vi "Dashboard Main.vi"() -> ()   [LabVIEW 2014]
uses:
  <vilib>/event_ctls.llb/eventvkey.ctl
  <vilib>/Rock Robotics/WPI/Dashboard/WPI_DashboardLogging Global.vi
  <vilib>/Utility/config.llb/Write Key (String).vi
  <vilib>/Utility/config.llb/Write Key (I32).vi
  Variables/Config_Global.vi
  <vilib>/Utility/config.llb/NI_LVConfig.lvlib
panel:
  out "error out 4":errorcluster
  out "error out 3":errorcluster
  out "error out 2":errorcluster
  out "error out":errorcluster
  in  "Rec Mode":enum32{"Stop", "Record", "Playback"}(radio)
  out "Camera Image":T1(plugin-control)
  out "Boolean":bool
  in  "TCP":refnum<k5>
  in  "Vision":u16(ring) items=["Camera Off", "USB Camera SW", "USB Camera HW", "IP Camera"]
  out "Camera IP":string
  out "Image Message":string="Timeout in Camera Communications"
  in  "Dashboard Tab":T2(tab)
  in  "Camera Settings":T3={"Frame Rate"=30, "Compression"=30, "Size"=1} {"Frame Rate" scale=1.0..30.0; "Size" items=["640x480", "320x240", "160x120"]}
  out "MotorChart R":cluster{"Numeric":dbl, "Numeric":dbl}(graph)
  out "MotorChart L":T4(graph)
  out "MotorSliders R":cluster{"MotorSlide1":dbl, "MotorSlide2":dbl} {"MotorSlide2" scale=-1.0..1.0 scale format="%#_2e"; "MotorSlide1" scale=-1.0..1.0 scale format="%#_2e"}
  out "MotorSliders L":T5 {"MotorSlide4 2" scale=0.0..14.0 scale format="%#_2e"; "MotorSlide2" scale=-1.0..1.0 scale format="%#_2e"; "MotorSlide1" scale=-1.0..1.0 scale format="%#_2e"}
  out "Gyro":dbl(knob) scale=0.0..360.0
  out "JS1 Z":dbl(slide) scale=-1.0..1.0 scale format="%#_2e"
  out "JS1 Graph":cluster{"X":dbl, "Y":dbl}[](graph)
  out "JS1 Buttons":T6
  out "JS2 Z":dbl(slide) scale=-1.0..1.0 scale format="%#_2e"
  out "JS2 Graph":cluster{"X":dbl, "Y":dbl}[](graph)
  out "JS2 Buttons":T6
  out "Mode":T7(ring)=enum."Auto Disabled"
  in  "DB Camera Config":bool
  out "fps":dbl format="%#.1g"
  out "Mbps":dbl format="%#.1g"
  out "Mbps 2":bool
  in  "DB/String 9":string
  in  "DB/String 8":string
  in  "DB/String 7":string
  in  "DB/String 6":string
  in  "DB/String 5":string
  in  "DB/String 4":string
  in  "DB/String 3":string
  in  "DB/String 2":string
  in  "DB/String 1":string
  in  "DB/String 0":string
  in  "DB/Slider 0":dbl(slide) scale=0.0..5.0
  in  "DB/Slider 1":dbl(slide) scale=0.0..5.0
  in  "DB/Slider 2":dbl(slide) scale=0.0..5.0
  in  "DB/Slider 3":dbl(slide) scale=0.0..5.0
  out "DB/LED 3":bool
  out "DB/LED 2":bool
  out "DB/LED 1":bool
  out "DB/LED 0":bool
  in  "DB/Button 3":bool
  in  "DB/Button 2":bool
  in  "DB/Button 1":bool
  in  "DB/Button 0":bool caption="New Name"
  in  "Test Slider":dbl(slide) scale=0.0..100.0 scale format="%#_3g"
  in  "On/Off":bool caption="Solenoid"
  in  "Test Name":u16(ring) items=["Select the test to run...", "Example Test", "-------------------------------", "List of tests is built in robot code.", "Replace with your own automated tests."]
  in  "Test Tree":string(tree)
  in  "Motor":cluster{"Value":dbl, "Enable":bool} {"Value" scale=-1.0..1.0 scale format="%#_3g"}
  out "Progress":T8 {"Test Progress" scale=0.0..100.0}
  in  "Rev/Fwd":cluster{"Forward":bool, "Reverse":bool}
  in  "Test Ring":u16(ring) items=["Monochrome", "Color"]
  in  "Listbox":i32(listbox)
  out "Tree":string(tree)
  in  "Tab Control 2":T9(tab)
  in  "Pod 0":T10
  in  "Pod 1":T10
  in  "Pod 2":T10
  in  "Pod 3":T10
  in  "General":T11
  out "error out":errorcluster
  # "Left"
  # "Front"
  # "Right"
  # "Battery"
  # "This tab is a great place for autonomous settings and robot-specific values.\nPlace controls and indicators inside this tab and match name to\nDashboard Variables on robot. You can also delete this comment."
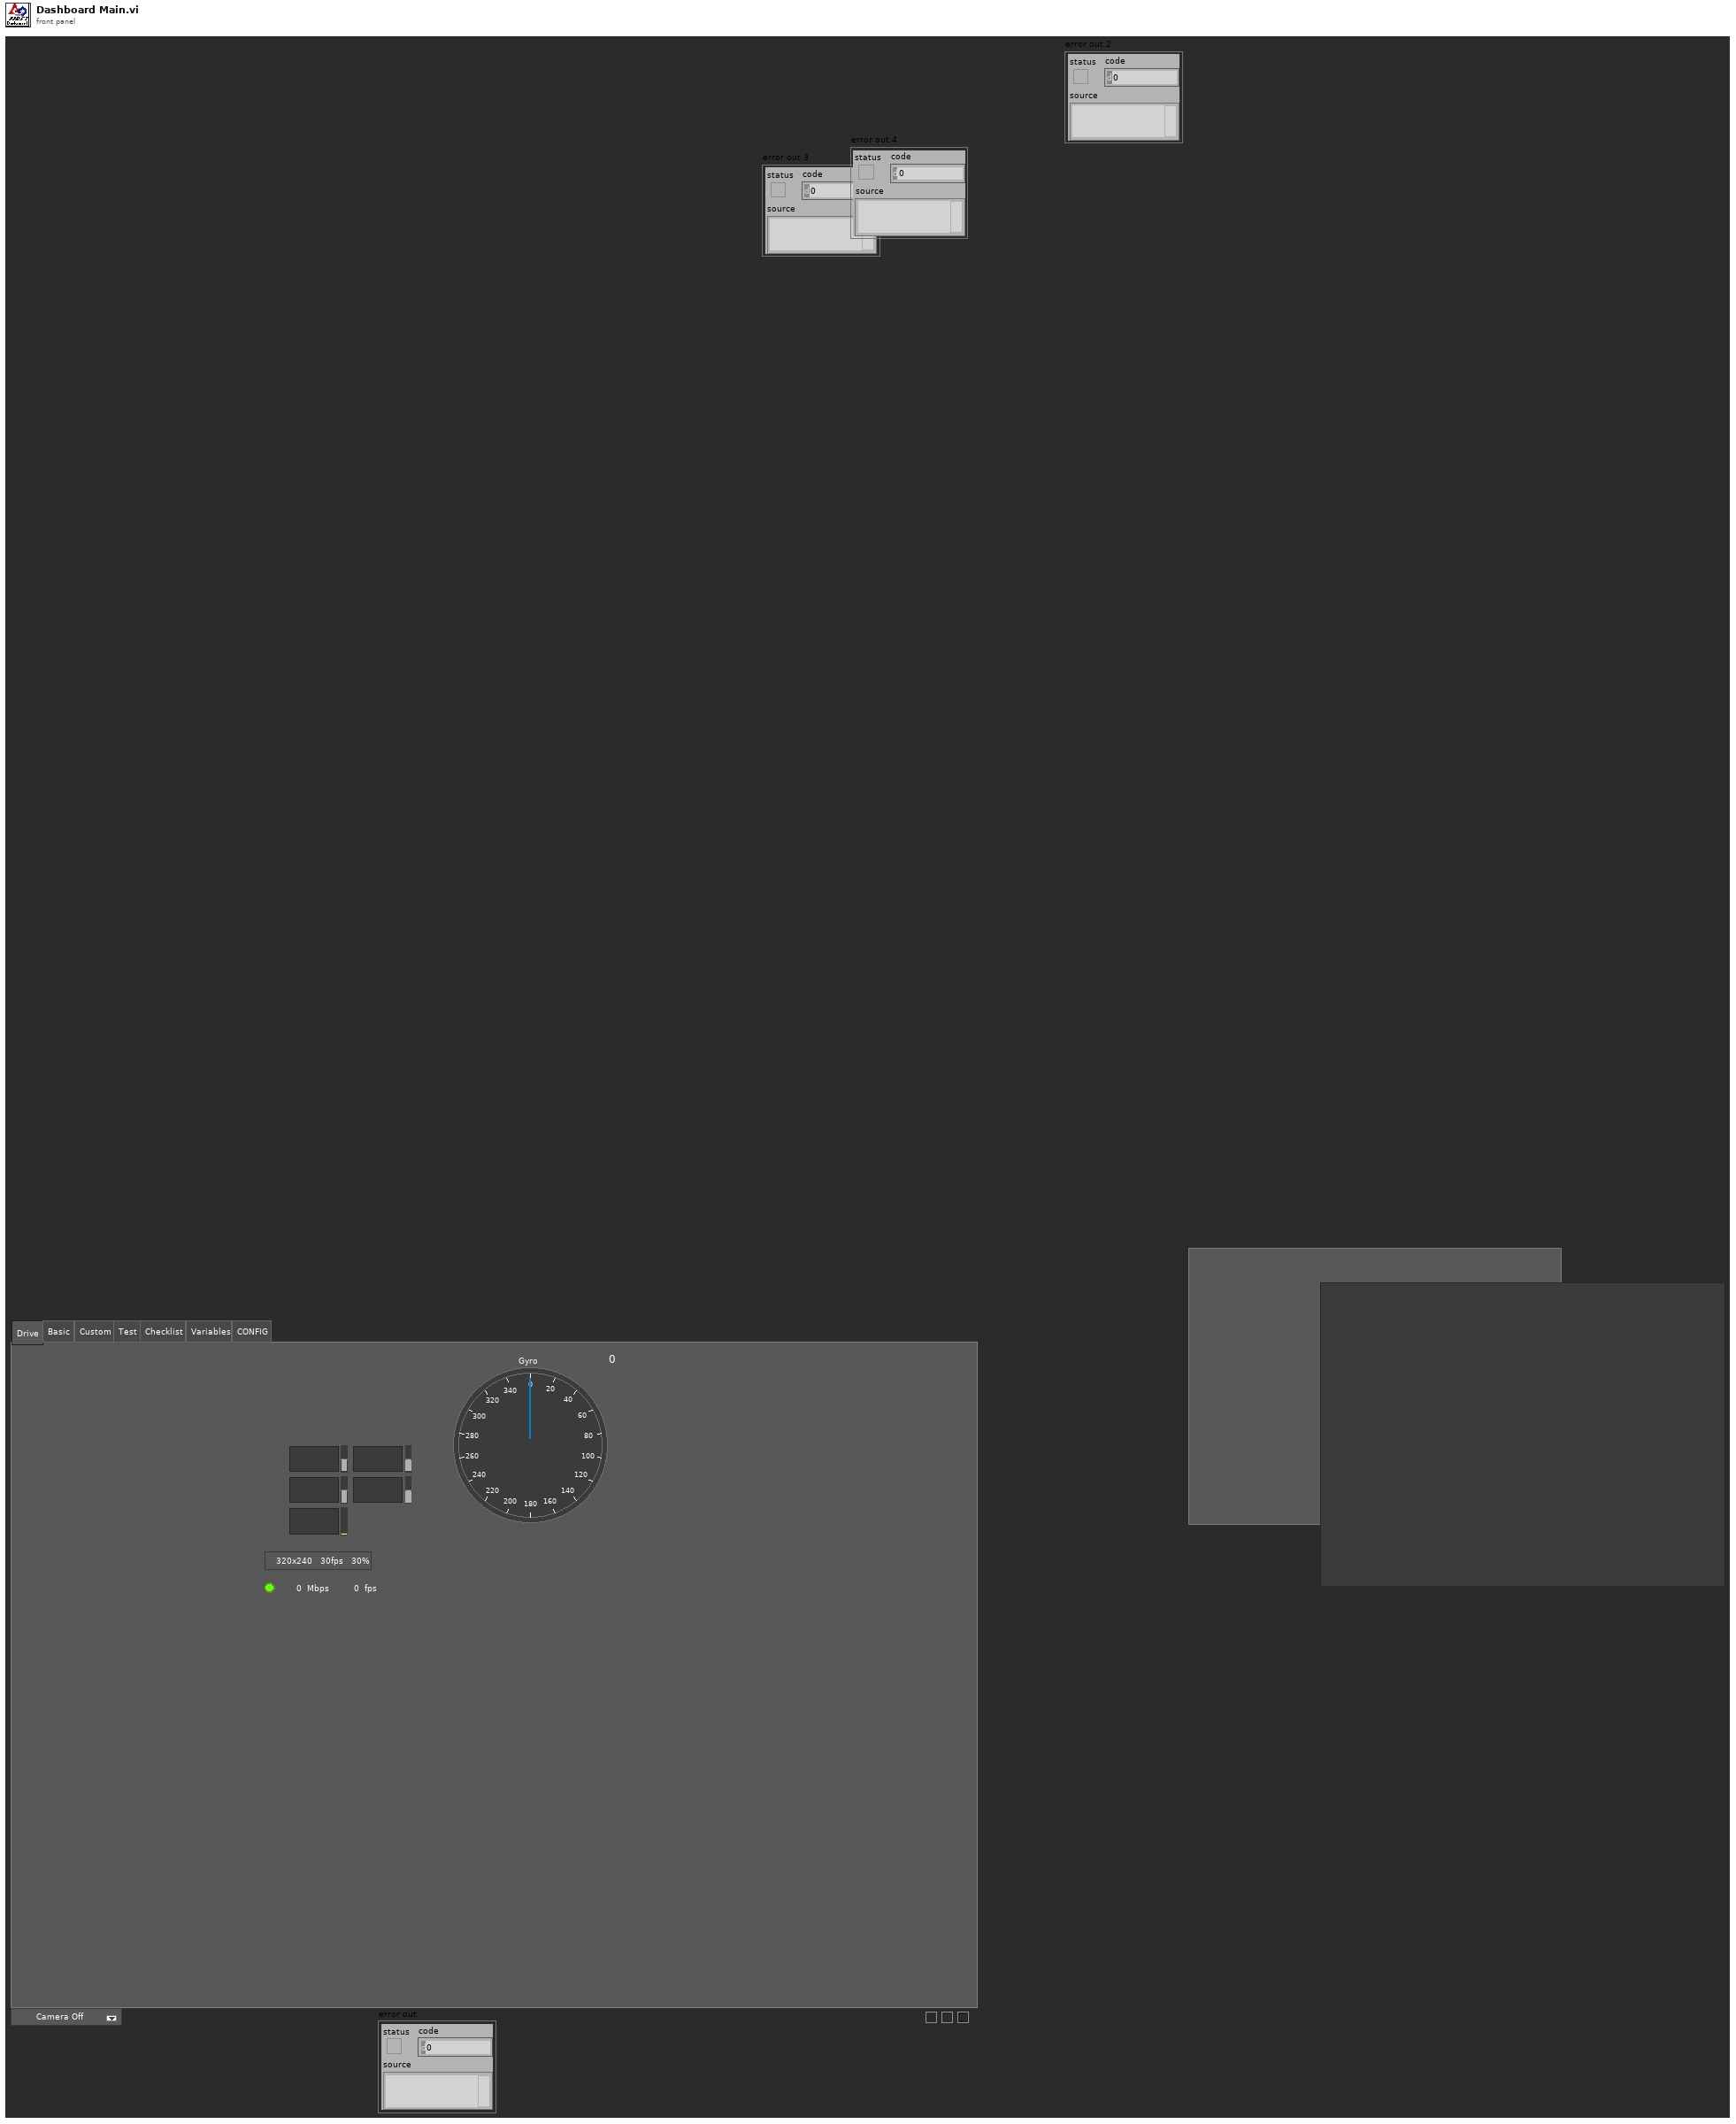
[diagram p1: front panel]
types:
  T1 = typedef "IMAQ Image.ctl" = refnum<image>
  T2 = enum32{"Drive", "Basic", "Custom", "Test", "Checklist", "Variables", "CONFIG"}
  T3 = cluster{"Frame Rate":i32, "Compression":i32, "Size":u16}
  T4 = cluster{"Numeric":dbl, "Numeric":dbl, "Battery V":dbl}
  T5 = cluster{"MotorSlide1":dbl, "MotorSlide2":dbl, "MotorSlide4 2":dbl}
  T6 = cluster{bool, bool, bool, bool, bool, bool, bool, bool, bool, bool, bool, bool}
  T7 = enum8{"Tele-Op Disabled", "Tele-Op Enabled", "Auto Disabled", "Auto Enabled", "Test Disabled", "Test Enabled", "Disconnected", "No Code", "E-Stop"}
  T8 = cluster{"Test Progress":u8, "Test Progress Text":string}
  T9 = enum32{"Pod 0", "Pod 1", "Pod 2", "Pod 3", "General"}
  T10 = cluster{"Drive":cluster{"DriveEncoder_CPfoot":dbl, "DriveEncoder_Location":string, "DriveEncoder_RoboRIO_PinA":i32, "DriveEncoder_RoboRIO_PinB":i32, "DriveEncoder_Invert?":bool, "DriverMotor_PID_P":dbl, "DriverMotor_PID_I":dbl, "DriverMotor_PID_D":dbl, "DriveMotor_CANorPWN_Channel":i32, "DriveMotor_Invert?":bool, "DriveMotor_IsCanSRX?":bool, "DriveMotor_MaxOutput":dbl, "DriveMotor_mINOutput":dbl}, "Turret":cluster{"TurretEncoder_Invert?":bool, "TurretEncoder_ZeroPosVolts":dbl, "TurretEncoder_Location":string, "TurretEncoder_RIO_AnalogChannel":dbl, "TurretMotor_Invert?":bool, "TurretMotor_PID_P":dbl, "TurretMotor_PID_I":dbl, "TurretMotor_PID_D":dbl, "TurretMotor_CANorPWN_Channel":dbl, "TurretMotor_IsCanSRX?":bool, "TurretMotor_MaxOutput?":dbl, "TurretMotor_MinOutput":dbl}, "Misc":cluster{"PodPosition_X":dbl, "PodPosition_Y":dbl, "PDP_Channel_Drive":i32, "PDP_Channel_Turret":i32}, "error out":errorcluster, "Warning":string}
  T11 = cluster{"PodCount":dbl, "PDP_CAN_ID":i32, "PCM_CAN_ID":i32, "BaseRobotMass":dbl, "Warning":string, "error out":errorcluster}
  T12 = enum32{"Drive", "Basic", "Custom", "Test", "Checklist", "Variables"}
  T13 = typedef "Image Type" = u32
  T14 = cluster{"Camera Image":refnum<vi>, "Dashboard Tab":refnum<vi>, "Boolean":refnum<vi>, "Vision":refnum<vi>, "Rec Mode":refnum<vi>, "Test Slider":refnum<vi>, "On/Off ":refnum<vi>, "Test Ring":refnum<vi>, "Rev/Fwd":refnum<vi>, "Test Name":refnum<vi>, "Motor":refnum<vi>, "Progress":refnum<vi>, "CheckList":refnum<vi>, "Tree":refnum<vi>, "Test Tree":refnum<vi>}
  T15 = cluster{"Error Strings":string, "Disable Counts":cluster{u16, u16}, "Rail Faults":cluster{u16, u16, u16}, "Robot IP":string, "DB Mode":u8, "Event Info":cluster{"Name":string, "Type":u8, "Number":u16, "Replay":u8}, "Camera Addr":string}
  T16 = cluster{"Storage":cluster{"Disk Free":u64, "RAM Block":u32, "RAM free":u32}, "CPU Utilization":cluster{"CPU % ISR":sgl, "CPU % Time Crit":sgl, "CPU % Timed Str":sgl, "CPU % High":sgl, "CPU % Above":sgl, "CPU % Normal":sgl, "CPU % Low":sgl}, "CAN":cluster{"% Bus Utilization":sgl, "Bus Off Cnt":u32, "TX_FIFO Full Cnt":u32, "Receive Error Cnt":u8, "Transmit Error Cnt":u8}, "HID":cluster{"HID Outputs":u32, "Rumble Low":u16, "Rumble High":u16}[]}
  T17 = cluster{"Status bits":cluster{"Test Mode":bool, "Autonomous":bool, "Enabled":bool, "Code Start":bool, "Brownout":bool, "Reserved 2":bool, "Reserved 3":bool, "E-Stop":bool}, "Code Trace":cluster{"Disabled":bool, "TeleOp":bool, "Auto":bool, "Test":bool}, "Controller Type":enum16{"unknown", "cRIO", "roboRio"}, "Code?":enum16{"unknown", "noCode", "code"}, "Battery V":dbl}
  T18 = cluster{"Control Bits":cluster{"TestMode":bool, "Autonomous":bool, "Enabled":bool, "FMS Present":bool, bool, bool, bool, "E-Stop":bool}, "Team Station ":u8, "Countdown":sgl, "Joystick Values":cluster{"Axes":dbl[], "Buttons":bool[], "POVs":i16[]}[]}
  T19 = cluster{"Axes":dbl[], "Buttons":bool[], "POVs":i16[]}[]
  T20 = cluster{"Axes":dbl[], "Buttons":bool[], "POVs":i16[]}
  T21 = cluster{"Buttons[0]":bool, "Buttons[1]":bool, "Buttons[2]":bool, "Buttons[3]":bool, "Buttons[4]":bool, "Buttons[5]":bool, "Buttons[6]":bool, "Buttons[7]":bool, "Buttons[8]":bool, "Buttons[9]":bool, "Buttons[10]":bool, "Buttons[11]":bool}
  T22 = typedef "NI_LVConfig.lvlib/Config Data RefNum.ctl" = refnum<k1>
  T23 = cluster{"Operation":enum16{"Update", "Clear"}, "Color Box":u32}[]
  T24 = typedef "eventvkey.ctl" = enum16{"ASCII", "Enter", "Return", "Shift", "Ctrl", "Alt", "Cmd", "Opt", "Caps", "NumLock", "Clear", "Break", "Up", "Down", "Left", "Right", "Insert", "Delete", "Home", "End", "PageUp", "PageDown", "Escape", "Help", "Pause", "ScrollLock", "F1", "F2", "F3", "F4", "F5", "F6", "F7", "F8", "F9", "F10", "F11", "F12", "F13", "F14", "F15", "F16", "F17", "F18", "F19", "F20", "F21", "F22", "F23", "F24", "Play", "VolumeUp", "VolumeDown", "Mute", "Two Byte Char"}
  T25 = cluster{"Image Size":bool, "Image Type":bool, "Pixel Value":bool, "ROI Information":bool, "Zoom Factor":bool}
  T26 = enum8{"Enabled", "Disabled", "Disabled and Grayed Out"}
  T27 = cluster{"Operation":enum16{"Update", "Clear"}, "Color Box":u32}
  T28 = cluster{"DriveEncoder_CPfoot":dbl, "DriveEncoder_Location":string, "DriveEncoder_RoboRIO_PinA":i32, "DriveEncoder_RoboRIO_PinB":i32, "DriveEncoder_Invert?":bool, "DriverMotor_PID_P":dbl, "DriverMotor_PID_I":dbl, "DriverMotor_PID_D":dbl, "DriveMotor_CANorPWN_Channel":i32, "DriveMotor_Invert?":bool, "DriveMotor_IsCanSRX?":bool, "DriveMotor_MaxOutput":dbl, "DriveMotor_mINOutput":dbl}
  T29 = cluster{"TurretEncoder_Invert?":bool, "TurretEncoder_ZeroPosVolts":dbl, "TurretEncoder_Location":string, "TurretEncoder_RIO_AnalogChannel":dbl, "TurretMotor_Invert?":bool, "TurretMotor_PID_P":dbl, "TurretMotor_PID_I":dbl, "TurretMotor_PID_D":dbl, "TurretMotor_CANorPWN_Channel":dbl, "TurretMotor_IsCanSRX?":bool, "TurretMotor_MaxOutput?":dbl, "TurretMotor_MinOutput":dbl}
  T30 = cluster{"PodPosition_X":dbl, "PodPosition_Y":dbl, "PDP_Channel_Drive":i32, "PDP_Channel_Turret":i32}
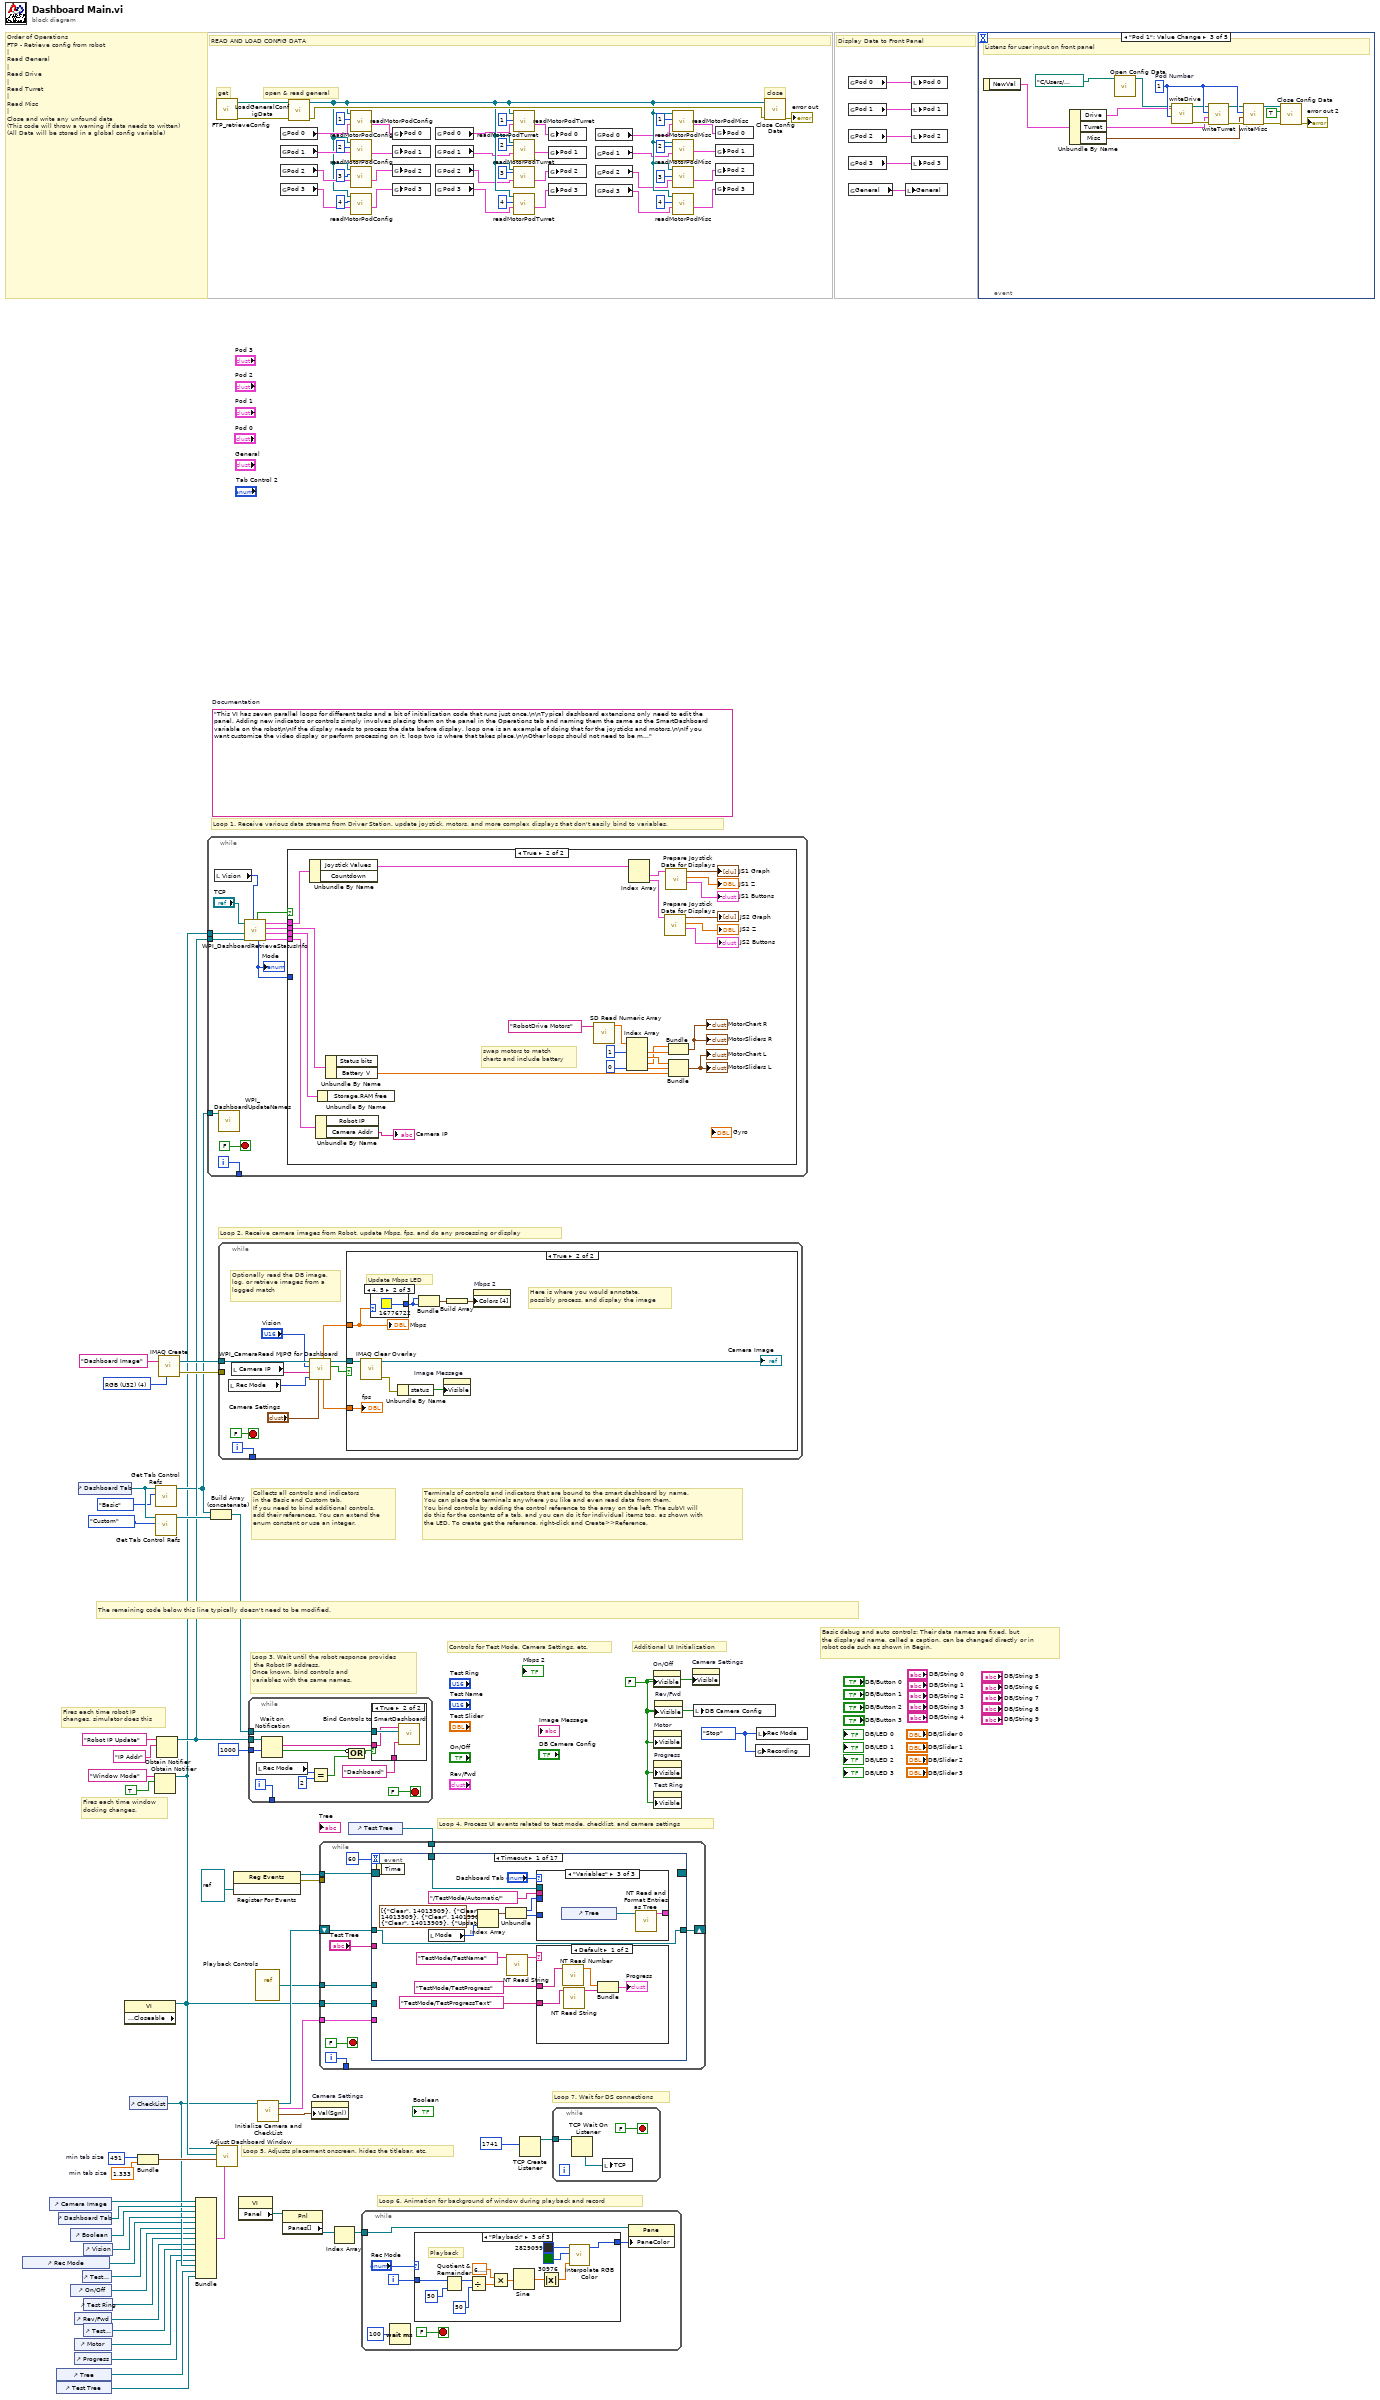
[diagram p0: block diagram]
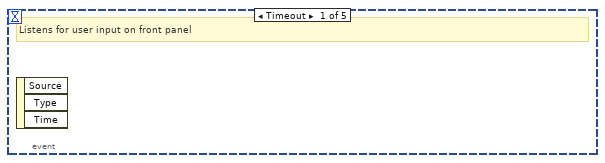
[diagram p2: hidden frame]
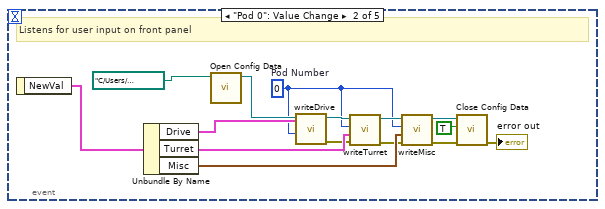
[diagram p3: hidden frame]
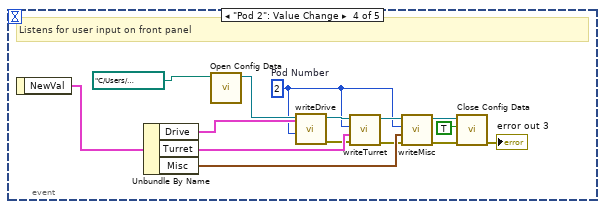
[diagram p4: hidden frame]
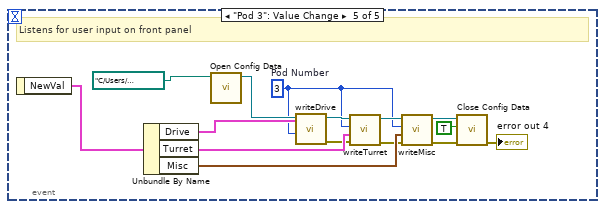
[diagram p5: hidden frame]
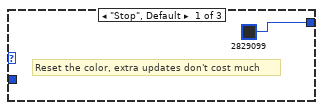
[diagram p7: hidden frame]
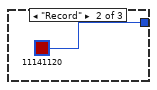
[diagram p8: hidden frame]
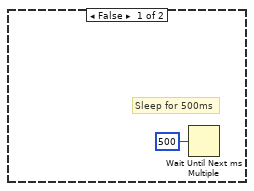
[diagram p10: hidden frame]
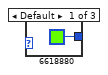
[diagram p11: hidden frame]
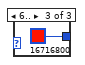
[diagram p12: hidden frame]
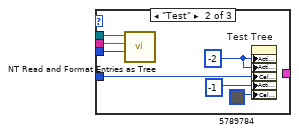
[diagram p14: hidden frame]
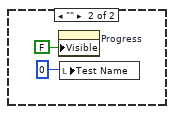
[diagram p15: hidden frame]
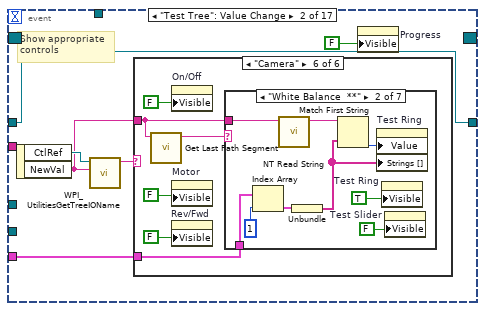
[diagram p16: hidden frame]
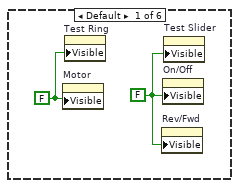
[diagram p17: hidden frame]
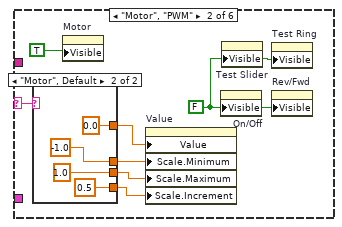
[diagram p18: hidden frame]
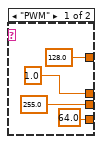
[diagram p19: hidden frame]
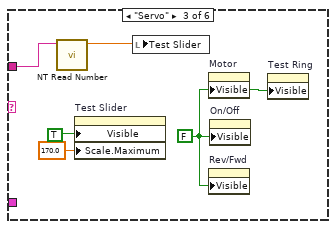
[diagram p20: hidden frame]
diagram:
  w70 = 491  # min tab size
  w69 = 1.333  # min tab size
  w78 = enum32{"Stop", "Record", "Playback"}."Stop" ("Rec Mode")
  w52 = FALSE ("Visible")
  (unwired) "This VI has seven parallel loops for different tasks and a bit of initialization code that runs just once.\n\nTypical dashboard extensions only need to edit the panel. Adding new indicators or controls simply involves placing them on the panel in the Operations tab and naming them the same as the SmartDashboard variable on the robot\n\nIf the display needs to process the data before display, loop one is an example of doing that for the joysticks and motors.\n\nIf you want customize the video display or perform processing on it, loop two is where that takes place.\n\nOther loops should not need to be modified. They are pretty standard, and document the task they perform."  # Documentation
  w98 = T13 4 items=["Grayscale (U8)", "Grayscale (I16)", "Grayscale (SGL)", "Complex (CSG)", "RGB (U32)", "HSL (U32)", "RGB (U64)"] ("Image Type")
  # "Display Data to Front Panel"
  # "Order of Operations\nFTP - Retrieve config from robot\n|\nRead General\n|\nRead Drive\n|\nRead Turret\n|\nRead Misc\n|\nClose and write any unfound data\n(This code will throw a warning if data needs to written)\n(All Data will be stored in a global config variable)"
  # "READ AND LOAD CONFIG DATA"
  # "open & read general"
  # "get"
  # "close"
  # "Loop 7. Wait for DS connections"
  # "Basic debug and auto controls: Their data names are fixed, but\nthe displayed name, called a caption, can be changed directly or in\nrobot code such as shown in Begin."
  # "Controls for Test Mode, Camera Settings, etc."
  # "Additional UI Initialization"
  # "Loop 6. Animation for background of window during playback and record"
  # "Fires each time robot IP\nchanges, simulator does this"
  # "Fires each time window\ndocking changes."
  # "Collects all controls and indicators\nin the Basic and Custom tab.\nIf you need to bind additional controls,\nadd their references. You can extend the\nenum constant or use an integer."
  # "The remaining code below this line typically doesn't need to be modified."
  # "Loop 4. Process UI events related to test mode, checklist, and camera settings"
  # "Terminals of controls and indicators that are bound to the smart dashboard by name.\nYou can place the terminals anywhere you like and even read data from them.\nYou bind controls by adding the control reference to the array on the left. The subVI will\ndo this for the contents of a tab, and you can do it for individual items too, as shown with\nthe LED. To create get the reference, right-click and Create>>Reference."
  # "Loop 3. Wait until the robot response provides\n the Robot IP address.\nOnce known, bind controls and\nvariables with the same names."
  # "Loop 5. Adjusts placement onscreen, hides the titlebar, etc."
  # "Loop 1. Receive various data streams from Driver Station, update joystick, motors, and more complex displays that don't easily bind to variables."
  # "Loop 2. Receive camera images from Robot, update Mbps, fps, and do any processing or display"
  n1 = control-ref of="Rec Mode"() -> (w58:refnum<vi>)
  n2 = control-ref of="Camera Image"() -> (w73:refnum<vi>)
  n3 = control-ref of="Tree"() -> (w62:refnum<vi>)
  n4 = control-ref of="Test Tree"() -> (w61:refnum<vi>)
  n5 = control-ref of="Dashboard Tab"() -> (w72:refnum<vi>)
  n6 = control-ref of="Boolean"() -> (w67:refnum<vi>)
  n7 = control-ref of="On/Off"() -> (w56:refnum<vi>)
  n8 = control-ref of="Progress"() -> (w53:refnum<vi>)
  n9 = control-ref of="Rev/Fwd"() -> (w54:refnum<vi>)
  n10 = control-ref of="Motor"() -> (w59:refnum<vi>)
  n11 = control-ref of="Dashboard Tab"() -> (w76:refnum<vi>)
  n12 = control-ref of="Test Slider"() -> (w57:refnum<vi>)
  n13 = control-ref of="Vision"() -> (w71:refnum<vi>)
  n14 = control-ref of="Test Ring"() -> (w55:refnum<vi>)
  n15 = control-ref of="Test Name"() -> (w60:refnum<vi>)
  n16 = property class="VI" props=["Front Panel.Closeable"]() -> (reference out=w77:refnum<vi>)  [unwired: 2 in, 2 out]
  n17 = control-ref of="CheckList"() -> (w63:refnum<vi>)
  n18 = Bundle("min tab size"=w70, "min tab size"=w69) -> (w68:cluster{"min tab size":i32, "min tab size":dbl})  [unwired: 1 in]
  n19 = Obtain Notifier(name (unnamed)="Window Mode", notification data type=TRUE) -> (notifier out=w49:refnum<notifier>)  [unwired: 2 in, 2 out]
  n20 = call <vilib>:"Get Tab Control Refs.vi"("Page Index"=T12."Basic" ("Dashboard Tab"), "TabControl in"=w76) -> ("ControlsOnPage"=w50:refnum<vi>[])  [unwired: 9 in]
  n21 = call <vilib>:"Get Tab Control Refs.vi"("Page Index"=T12."Custom" ("Dashboard Tab"), "TabControl in"=w76) -> ("ControlsOnPage"=w75:refnum<vi>[])  [unwired: 9 in]
  n22 = Obtain Notifier(name (unnamed)="Robot IP Update", notification data type="IP Addr" ("name (unnamed)")) -> (notifier out=w51:refnum<notifier>)  [unwired: 2 in, 2 out]
  n23 = call "IMAQ Create"("Image Name"="Dashboard Image", "Image Type"=w98) -> ("New Image"=w96:T1, "error out"=w95:errorcluster)  [unwired: 2 in, 1 out]
  n24 = Bundle("Camera Image"=w73, "Dashboard Tab"=w72, "Boolean"=w67, "Vision"=w71, "Rec Mode"=w58, "Test Slider"=w57, "On/Off"=w56, "Test Ring"=w55, "Rev/Fwd"=w54, "Test Name"=w60, "Motor"=w59, "Progress"=w53, "CheckList"=w63, "Tree"=w62, "Test Tree"=w61) -> (w64:T14)  [unwired: 1 in]
  n25 = while {
    tunnel: [w110] -> _
    tunnel: w51 -> [w104]
    tunnel: w50 -> [w103]
    tunnel: w49 -> [w99]
    i -> [w110]
    stop <- FALSE stop-if-true
    n26 = local read "Vision"() -> (w101:u16)
    n27 = call <vilib>:"WPI_DashboardUpdateNames.vi"("Controls on Tab"=w103) -> ()  [unwired: 11 in]
    n28 = call <vilib>:"WPI_DashboardRetrieveStatusInfo.vi"("Vision"=w101, "Binding Refnum"=w104, "Window Mode Notifier"=w99, "TCP Cnx"="TCP") -> ("Power and Errors"=w105:T15, "Robot Metrics"=w108:T16, "Status Info"=w109:T17, "Control Info"=w106:T18, "Robot Mode"=w102:T7, "Process?"=w107:bool)  [unwired: 2 in]
    "Mode" <- w102
    n29 = case shown="True" w107 {
      tunnel: w109 -> [_ w136]
      tunnel: w108 -> [_ w135]
      tunnel: w106 -> [_ w134]
      tunnel: w105 -> [_ w133]
      tunnel: w102 -> [_ _]
      frame False {
      }
      frame True {
        # "swap motors to match\ncharts and include battery"
        n30 = Unbundle By Name(w134) -> ("Joystick Values"=w121:T19)  [unwired: 1 out]
        n31 = Unbundle By Name(w133) -> ("Camera Addr"=→"Camera IP":string)  [unwired: 1 out]
        n32 = Unbundle By Name(w135) -> ()  [unwired: 1 out]
        n33 = Unbundle By Name(w136) -> ("Battery V"=w122:dbl)  [unwired: 1 out]
        n34 = call <vilib>:"SD Read Numeric Array.vi"("Name"="RobotDrive Motors") -> ("Numeric Array"=w124:dbl[])  [unwired: 8 in, 2 out]
        n35 = Index Array(array=w124, index #1=1, index #4=0) -> (element #1=w128:dbl, element #2=w129:dbl, element #3=w127:dbl, element #4=w132:dbl)  [unwired: 2 in]
        n36 = Index Array(array=w121) -> (element #1=w120:T20, element #2=w115:T20)  [unwired: 2 in]
        n37 = call "Prepare Joystick Data for Displays.vi"("Joystick Values"=w115) -> ("Buttons"=→"JS2 Buttons":T21, "Z Axis"=→"JS2 Z":dbl, "Cartesian Data"=→"JS2 Graph":cluster{"X axis":dbl, "X axis":dbl}[])  [unwired: 8 in]
        n38 = call "Prepare Joystick Data for Displays.vi"("Joystick Values"=w120) -> ("Buttons"=→"JS1 Buttons":T21, "Z Axis"=→"JS1 Z":dbl, "Cartesian Data"=→"JS1 Graph":cluster{"X axis":dbl, "X axis":dbl}[])  [unwired: 8 in]
        n39 = Bundle("Numeric"=w127, "Numeric"=w128) -> (→"MotorChart R" →"MotorSliders R":cluster{"Numeric":dbl, "Numeric":dbl})  [unwired: 1 in]
        n40 = Bundle("Numeric"=w129, "Numeric"=w132, "Battery V"=w122) -> (→"MotorChart L" →"MotorSliders L":T4)  [unwired: 1 in]
      }
    }
  }
  n41 = Build Array (concatenate)(w50, w75) -> (w74:refnum<vi>[])
  n42 = call "FTP_retrieveConfig.vi"() -> ("error out"=w45:errorcluster, "local path"=w46:path)  [unwired: 10 in]
  n43 = call "Adjust Dashboard Window.vi"("Sizing Refnums"=w64, "Size Constraints"=w68, "VI"=w77, "Notifier in"=w49) -> ()  [unwired: 8 in]
  n44 = while {
    tunnel: w96 -> [w145]
    tunnel: w95 -> [_]
    tunnel: [w146] -> _
    i -> [w146]
    stop <- FALSE stop-if-true
    # "Optionally read the DB image,\nlog, or retrieve images from a\nlogged match"
    n45 = local read "Rec Mode"() -> (w139:enum32{"Stop", "Record", "Playback"})
    n46 = local read "Camera IP"() -> (w137:string)
    n47 = call <vilib>:"WPI_CameraRead MJPG for Dashboard.vi"("Camera Settings"="Camera Settings", "Rec Mode"=w139, "Camera IP"=w137, "Camera Mode"="Vision", "Refnum in"=w145) -> ("Active"=w143:bool, "Refnum out"=w144:T1, "FPS"=w142:dbl, "Bandwidth (Mbps)"=w141:dbl)  [unwired: 3 in]
    n48 = case shown="True" w143 {
      tunnel: w144 -> [_ w152]
      tunnel: w141 -> [_ w151]
      tunnel: w142 -> [_ w149]
      frame False {
        # "Sleep for 500ms"
        n49 = Wait Until Next ms Multiple(millisecond multiple=u32 500) -> ()  [unwired: 1 out]
      }
      frame True {
        # "Here is where you would annotate,\npossibly process, and display the image"
        # "Update Mbps LED"
        n50 = call "IMAQ Clear Overlay"("Image"=w152) -> ("error out"=w156:errorcluster, "Image Out"=→"Camera Image":T1)  [unwired: 2 in, 7 out]
        n51 = case shown="4, 5" w151 {
          tunnel: [u32 6618880 ("Color Box") u32 16776722 ("Color Box") u32 16716800 ("Color Box")] -> w153
          frame Default {
          }
          frame 4, 5 {
          }
          frame 6.. {
          }
        }
        n52 = Unbundle By Name(w156) -> ("status"=w157:bool)
        n53 = Bundle("Color Box"=w153, "Color Box"=w153) -> (w155:cluster{"Color Box":u32, "Color Box":u32})  [unwired: 1 out]
        n54 = property on="Image Message" class="Str"("Visible"=w157) -> ()  [unwired: 2 in, 2 out]
        n55 = Build Array(w155) -> (w154:cluster{"Color Box":u32, "Color Box":u32}[])
        n56 = property on="Mbps 2" class="Bool (strict)"("Colors [4]"=w154) -> ()  [unwired: 2 in, 2 out]
        "Mbps" <- w151
        "fps" <- w149
      }
    }
  }
  n57 = register-events(refnum<vi> refnum) -> (reference out=w82:refnum<event-registration>, error out=w81:errorcluster)  [unwired: 2 in]
  n58 = property class="VI"() -> ("Panel"=w85:refnum<vi>)  [unwired: 2 in, 2 out]
  n59 = while {
    tunnel: w74 -> [w172]
    tunnel: w51 -> [w170]
    tunnel: [w168] -> _
    tunnel: u32 1000 ("milliseconds to wait") -> [w167]
    i -> [w168]
    stop <- FALSE stop-if-true
    n60 = local read "Rec Mode"() -> (w163:enum32{"Stop", "Record", "Playback"})
    n61 = Wait on Notification(notifier=w170, timeout in ms (-1)=w167) -> (notification=w169:string, timed out?=w165:bool)  [unwired: 2 in, 2 out]
    n62 = Equal?(x=w163, y=u16 2 ("Rec Mode")) -> (x = y?=w164:bool)
    n63 = Compound Arithmetic op=OR(invert w165, w164) -> (w166:bool)
    n64 = case shown="True" w166 {
      tunnel: w172 -> [_ w175]
      tunnel: w169 -> [_ w174]
      tunnel: "Dashboard" -> [_ w173]
      frame False {
      }
      frame True {
        n65 = call <vilib>:"Bind Controls to SmartDashboard.vi"("Client Name"=w173, "Bound Control Refs"=w175, "Server IP Address"=w174) -> ()  [unwired: 9 in]
      }
    }
  }
  n66 = vi-ref "Playback Controls.vi"() -> (w83:refnum<vi>)
  n67 = call "Initialize Camera and CheckList.vi"("ListBox in"=w63) -> ("Cluster"=w89:cluster{"value":i32, "value":i32, "index":i32}, "Array"=w90:cluster{string[]}[], "File Refnum"=w88:T22)  [unwired: 8 in]
  n68 = global read "Config_Global.vi" "Pod 0"() -> (w31:T10)
  n69 = global read "Config_Global.vi" "Pod 1"() -> (w30:T10)
  n70 = global read "Config_Global.vi" "Pod 2"() -> (w29:T10)
  n71 = global read "Config_Global.vi" "Pod 3"() -> (w28:T10)
  n72 = property class="Pnl"(reference=w85) -> ("Panes[]"=w86:refnum<vi>[])  [unwired: 1 in, 2 out]
  n73 = call "LoadGeneralConfigData.vi"("error in (no error)"=w45, "configuration file path"=w46) -> ("error out"=w23:errorcluster, "Refnum out"=w22:T22)  [unwired: 8 in]
  n74 = property on="Camera Settings" class="Clust (strict)"("Val(Sgnl)"=w89) -> ()  [unwired: 2 in, 2 out]
  n75 = Index Array(array=w86) -> (element=w84:refnum<vi>)  [unwired: 1 in]
  n76 = control-ref of="Test Tree"() -> (w87:refnum<vi>)
  n77 = while {
    tunnel: w90 -> [w183]
    shift-right: [w182] -> _
    shift-left: w88 -> [w181]
    tunnel: [w180] -> _
    tunnel: w87 -> [w179]
    tunnel: w83 -> [w178]
    tunnel: w82 -> [w177]
    tunnel: w81 -> [_]
    tunnel: w77 -> [w176]
    i -> [w180]
    stop <- FALSE stop-if-true
    n78 = event shown="[0] Timeout" {
      selector: w177 -> [_ _ _ _ _ _ _ _ _ _ _ _ _ _ _ _ _]
      dyn-events: [_ _ _ _ _ _ _ _ _ _ _ _ _ w421 _ _ _] -> _
      timeout: u32 60 ("milliseconds to wait") -> [_ _ _ _ _ _ _ _ _ _ _ _ _ _ _ _ _]
      tunnel: w179 -> [w195 _ _ _ _ _ _ _ _ _ _ _ _ _ _ _ _]
      tunnel: "Test Tree" -> [_ _ _ _ _ _ _ _ w390 w398 w400 w404 w412 _ _ _ _]
      tunnel: w183 -> [_ w217 _ _ _ _ w354 w384 _ _ _ _ _ _ _ _ _]
      tunnel: [w191 w216 w315 w320 w328 w340 w353 w377 w389 w396 w399 w403 w411 w423 w437 w438 w448] -> w182
      tunnel: w181 -> [w191 w216 w315 w320 w328 w340 w352 w377 w389 w396 w399 w403 w411 w423 w437 w438 w448]
      tunnel: w178 -> [_ _ _ _ _ _ _ _ _ _ _ _ _ w424 _ w441 _]
      tunnel: w176 -> [_ _ _ _ _ _ _ _ _ _ _ _ _ w419 _ _ _]
      event Timeout {
        n79 = event-data() -> ()  [unwired: 1 in, 1 out]
        n80 = local read "Mode"() -> (w194:T7)
        n81 = Index Array(array=T23 [{"Operation"=enum."Clear", "Color Box"=14013909}, {"Operation"=enum."Clear", "Color Box"=14013909}, {"Operation"=enum."Clear", "Color Box"=14013909}, {"Operation"=enum."Clear", "Color Box"=14013909}, {"Operation"=enum."Update", "Color Box"=14013909}, {"Operation"=enum."Update", "Color Box"=16777215}, {"Operation"=enum."Clear", "Color Box"=14013909}, {"Operation"=enum."Clear", "Color Box"=14013909}, {"Operation"=enum."Clear", "Color Box"=14013909}], index=w194) -> (element=w189:T27)
        n82 = Unbundle(w189) -> ("Operation"=w188:enum16{"Update", "Clear"}, "Color Box"=w187:u32)
        n83 = call <vilib>:"NT Read String.vi"("Name"="TestMode/TestName") -> ("String"=w198:string)  [unwired: 9 in, 1 out]
        n84 = case shown="\"Variables\"" "Dashboard Tab" {
          tunnel: w195 -> [_ w206 _]
          tunnel: "/TestMode/Automatic/" ("Name Pattern") -> [_ w205 _]
          tunnel: w188 -> [_ w204 _]
          tunnel: [_ _ w208] -> _
          tunnel: w187 -> [_ w200 _]
          frame "Custom", Default {
          }
          frame "Test" {
            w203 = -2 ("Active Item:Row Number")
            n85 = call <vilib>:"NT Read and Format Entries as Tree.vi"("Operation"=w204, "Name Pattern"=w205, "Tree Refnum"=w206) -> ()  [unwired: 7 in, 2 out]
            n86 = property on="Test Tree" class="Tree (strict)"("Active Item Row Number"=w203, "ActiveColNum"=w203, "CellBG"=w200, "Active Item Row Number"=-1 ("Active Item:Row Number"), "CellBG"=u32 5789784 ("Color Box")) -> ()  [unwired: 2 in, 2 out]
          }
          frame "Variables" {
            n87 = control-ref of="Tree"() -> (w207:refnum<vi>)
            n88 = call <vilib>:"NT Read and Format Entries as Tree.vi"("Tree Refnum"=w207) -> ("Formatted Strings"=w208:cluster{"Name":string, "Value":string}[])  [unwired: 9 in, 1 out]
          }
        }
        n89 = case shown="Default" w198 {
          tunnel: "TestMode/TestProgress" ("Name") -> [w210 _]
          tunnel: "TestMode/TestProgressText" ("Name") -> [w209 _]
          frame Default {
            n90 = call <vilib>:"NT Read Number.vi"("Name"=w210) -> ("Numeric"=w211:dbl)  [unwired: 9 in, 1 out]
            n91 = call <vilib>:"NT Read String.vi"("Name"=w209) -> ("String"=w212:string)  [unwired: 9 in, 1 out]
            n92 = Bundle("Numeric"=w211, "String"=w212) -> (→"Progress":cluster{"Numeric":dbl, "String":string})  [unwired: 1 in]
          }
          frame "" {
            n93 = property on="Progress" class="Clust (strict)"("Visible"=FALSE) -> ()  [unwired: 2 in, 2 out]
            n94 = local write "Test Name"(u16 0) -> ()
          }
        }
      }
      event "Test Tree": Value Change {
        # "Show appropriate\ncontrols"
        n95 = event-data() -> ("CtlRef"=w220:refnum<vi>, "NewVal"=w218:string)  [unwired: 1 in]
        n96 = call <vilib>:"WPI_UtilitiesGetTreeIOName.vi"("NewVal"=w218, "TreeControl in"=w220) -> ("I/O Name"=w221:string)  [unwired: 9 in]
        n97 = case shown="\"Camera\"" w221 {
          selector: w221 -> [_ w228 _ w246 w255 _]
          tunnel: w218 -> [_ _ w243 w245 _ w262]
          tunnel: w217 -> [_ _ _ _ _ w261]
          frame Default {
            w223 = FALSE ("Visible")
            w222 = FALSE ("Visible")
            n98 = property on="Motor" class="Clust (strict)"("Visible"=w222) -> ()  [unwired: 2 in, 2 out]
            n99 = property on="Test Ring" class="Ring (strict)"("Visible"=w222) -> ()  [unwired: 2 in, 2 out]
            n100 = property on="Rev/Fwd" class="Clust (strict)"("Visible"=w223) -> ()  [unwired: 2 in, 2 out]
            n101 = property on="On/Off" class="Bool (strict)"("Visible"=w223) -> ()  [unwired: 2 in, 2 out]
            n102 = property on="Test Slider" class="Slide (strict)"("Visible"=w223) -> ()  [unwired: 2 in, 2 out]
          }
          frame "Motor", "PWM" {
            w229 = FALSE ("Visible")
            n103 = case shown="\"Motor\", Default" w228 {
              tunnel: [1.0 ("Value") -1.0 ("Value")] -> w227
              tunnel: [255.0 ("Value") 1.0 ("Value")] -> w226
              tunnel: [128.0 ("Value") 0.0 ("Value")] -> w225
              tunnel: [64.0 ("Value") 0.5 ("Value")] -> w224
              frame "PWM" {
              }
              frame "Motor", Default {
              }
            }
            n104 = property on="Motor" class="Clust (strict)"("Visible"=TRUE) -> ()  [unwired: 2 in, 2 out]
            n105 = property on="Value" class="Slide (strict)"("Value"=w225, "Scale.Minimum"=w227, "Scale.Maximum"=w226, "Scale.Increment"=w224) -> ()  [unwired: 2 in, 2 out]
            n106 = property on="On/Off" class="Bool (strict)"("Visible"=w229) -> ()  [unwired: 2 in, 2 out]
            n107 = property on="Test Slider" class="Slide (strict)"("Visible"=w229) -> ()  [unwired: 2 in, 2 out]
            n108 = property on="Test Ring" class="Ring (strict)"("Visible"=w229) -> ()  [unwired: 2 in, 2 out]
            n109 = property on="Rev/Fwd" class="Clust (strict)"("Visible"=w229) -> ()  [unwired: 2 in, 2 out]
          }
          frame "Servo" {
            w241 = FALSE ("Visible")
            n110 = call <vilib>:"NT Read Number.vi"("Name"=w243) -> ("Numeric"=w242:dbl)  [unwired: 9 in, 1 out]
            n111 = property on="Test Slider" class="Slide (strict)"("Visible"=TRUE, "Scale.Maximum"=170.0 ("Scale.Range:Maximum")) -> ()  [unwired: 2 in, 2 out]
            n112 = local write "Test Slider"(w242) -> ()
            n113 = property on="Motor" class="Clust (strict)"("Visible"=w241) -> ()  [unwired: 2 in, 2 out]
            n114 = property on="Rev/Fwd" class="Clust (strict)"("Visible"=w241) -> ()  [unwired: 2 in, 2 out]
            n115 = property on="On/Off" class="Bool (strict)"("Visible"=w241) -> ()  [unwired: 2 in, 2 out]
            n116 = property on="Test Ring" class="Ring (strict)"("Visible"=w241) -> ()  [unwired: 2 in, 2 out]
          }
          frame "Relay", "Solenoid" {
            w244 = FALSE ("Visible")
            n117 = property on="Motor" class="Clust (strict)"("Visible"=w244) -> ()  [unwired: 2 in, 2 out]
            n118 = property on="Test Slider" class="Slide (strict)"("Visible"=w244) -> ()  [unwired: 2 in, 2 out]
            n119 = Search and Replace String(input string=w245, search string="/Value  **", replace string="/Direction") -> (result string=w251:string)  [unwired: 5 in, 3 out]
            n120 = property on="Test Ring" class="Ring (strict)"("Visible"=w244) -> ()  [unwired: 2 in, 2 out]
            n121 = call <vilib>:"NT Read String.vi"("Name"=w251) -> ("String"=w249:string)  [unwired: 9 in, 1 out]
            n122 = Equal?(x="Both directions", y=w249) -> (x = y?=w247:bool)
            n123 = Not(x=w247) -> (.not. x?=w248:bool)
            n124 = property on="Rev/Fwd" class="Clust (strict)"("Visible"=w247) -> ()  [unwired: 2 in, 2 out]
            n125 = property on="On/Off" class="Bool (strict)"("Visible"=w248, "Caption.Text"=w246) -> ()  [unwired: 2 in, 2 out]
          }
          frame "Compressor", "Digital Out" {
            w254 = FALSE ("Visible")
            # "Get direction and finish"
            n126 = property on="Motor" class="Clust (strict)"("Visible"=w254) -> ()  [unwired: 2 in, 2 out]
            n127 = property on="Test Slider" class="Slide (strict)"("Visible"=w254) -> ()  [unwired: 2 in, 2 out]
            n128 = property on="Test Ring" class="Ring (strict)"("Visible"=w254) -> ()  [unwired: 2 in, 2 out]
            n129 = property on="On/Off" class="Bool (strict)"("Visible"=TRUE, "Caption.Text"=w255) -> ()  [unwired: 2 in, 2 out]
            n130 = property on="Rev/Fwd" class="Clust (strict)"("Visible"=FALSE) -> ()  [unwired: 2 in, 2 out]
          }
          frame "Camera" {
            n131 = call <vilib>:"Get Last Path Segment.vi"("String in"=w262) -> ("String out"=w263:string)  [unwired: 10 in]
            n132 = property on="On/Off" class="Bool (strict)"("Visible"=FALSE) -> ()  [unwired: 2 in, 2 out]
            n133 = property on="Motor" class="Clust (strict)"("Visible"=FALSE) -> ()  [unwired: 2 in, 2 out]
            n134 = property on="Rev/Fwd" class="Clust (strict)"("Visible"=FALSE) -> ()  [unwired: 2 in, 2 out]
            n135 = case shown="\"White Balance  **\"" w263 {
              tunnel: w262 -> [w269 w278 w287 w296 w305 _ w311]
              tunnel: w261 -> [w267 w275 w284 w293 w302 _ _]
              frame "Size  **" {
                n136 = Index Array(array=w267) -> (element=w266:cluster{string[]})  [unwired: 1 in]
                n137 = call <vilib>:"NT Read String.vi"("Name"=w269) -> ("String"=w268:string)  [unwired: 9 in, 1 out]
                n138 = Unbundle(w266) -> (w264:string[])
                n139 = Match First String(2:w264, 3:w268) -> (0:w265:i32)  [unwired: 1 out]
                n140 = property on="Test Ring" class="Ring (strict)"("Value"=w265, "Strings []"=w264) -> ()  [unwired: 2 in, 2 out]
                n141 = property on="Test Ring" class="Ring (strict)"("Visible"=TRUE) -> ()  [unwired: 2 in, 2 out]
                n142 = property on="Test Slider" class="Slide (strict)"("Visible"=FALSE) -> ()  [unwired: 2 in, 2 out]
              }
              frame "White Balance  **" {
                n143 = Index Array(array=w275, index=1) -> (element=w276:cluster{string[]})
                n144 = call <vilib>:"NT Read String.vi"("Name"=w278) -> ("String"=w277:string)  [unwired: 9 in, 1 out]
                n145 = Unbundle(w276) -> (w273:string[])
                n146 = Match First String(2:w273, 3:w277) -> (0:w272:i32)  [unwired: 1 out]
                n147 = property on="Test Ring" class="Ring (strict)"("Value"=w272, "Strings []"=w273) -> ()  [unwired: 2 in, 2 out]
                n148 = property on="Test Ring" class="Ring (strict)"("Visible"=TRUE) -> ()  [unwired: 2 in, 2 out]
                n149 = property on="Test Slider" class="Slide (strict)"("Visible"=FALSE) -> ()  [unwired: 2 in, 2 out]
              }
              frame "Exposure  **" {
                n150 = Index Array(array=w284, index=2) -> (element=w285:cluster{string[]})
                n151 = call <vilib>:"NT Read String.vi"("Name"=w287) -> ("String"=w286:string)  [unwired: 9 in, 1 out]
                n152 = Unbundle(w285) -> (w281:string[])
                n153 = Match First String(2:w281, 3:w286) -> (0:w282:i32)  [unwired: 1 out]
                n154 = property on="Test Ring" class="Ring (strict)"("Value"=w282, "Strings []"=w281) -> ()  [unwired: 2 in, 2 out]
                n155 = property on="Test Ring" class="Ring (strict)"("Visible"=TRUE) -> ()  [unwired: 2 in, 2 out]
                n156 = property on="Test Slider" class="Slide (strict)"("Visible"=FALSE) -> ()  [unwired: 2 in, 2 out]
              }
              frame "Exposure Priority  **" {
                n157 = Index Array(array=w293, index=3) -> (element=w294:cluster{string[]})
                n158 = call <vilib>:"NT Read String.vi"("Name"=w296) -> ("String"=w295:string)  [unwired: 9 in, 1 out]
                n159 = Unbundle(w294) -> (w290:string[])
                n160 = Match First String(2:w290, 3:w295) -> (0:w291:i32)  [unwired: 1 out]
                n161 = property on="Test Ring" class="Ring (strict)"("Value"=w291, "Strings []"=w290) -> ()  [unwired: 2 in, 2 out]
                n162 = property on="Test Ring" class="Ring (strict)"("Visible"=TRUE) -> ()  [unwired: 2 in, 2 out]
                n163 = property on="Test Slider" class="Slide (strict)"("Visible"=FALSE) -> ()  [unwired: 2 in, 2 out]
              }
              frame "Color Enable  **" {
                n164 = Index Array(array=w302, index=4) -> (element=w303:cluster{string[]})
                n165 = call <vilib>:"NT Read String.vi"("Name"=w305) -> ("String"=w304:string)  [unwired: 9 in, 1 out]
                n166 = Unbundle(w303) -> (w299:string[])
                n167 = Match First String(2:w299, 3:w304) -> (0:w300:i32)  [unwired: 1 out]
                n168 = property on="Test Ring" class="Ring (strict)"("Value"=w300, "Strings []"=w299) -> ()  [unwired: 2 in, 2 out]
                n169 = property on="Test Ring" class="Ring (strict)"("Visible"=TRUE) -> ()  [unwired: 2 in, 2 out]
                n170 = property on="Test Slider" class="Slide (strict)"("Visible"=FALSE) -> ()  [unwired: 2 in, 2 out]
              }
              frame Default {
                n171 = property on="Test Ring" class="Ring (strict)"("Visible"=FALSE) -> ()  [unwired: 2 in, 2 out]
                n172 = property on="Test Slider" class="Slide (strict)"("Visible"=FALSE) -> ()  [unwired: 2 in, 2 out]
              }
              frame "Brightness  **", "Color Level  **", "Compression  **", "FPS  **", "Sharpness  **" {
                n173 = call <vilib>:"NT Read Number.vi"("Name"=w311) -> ("Numeric"=w310:dbl)  [unwired: 9 in, 1 out]
                n174 = local write "Test Slider"(w310) -> ()
                n175 = property on="Test Slider" class="Slide (strict)"("Visible"=TRUE, "Scale.Maximum"=100.0 ("Scale.Range:Maximum")) -> ()  [unwired: 2 in, 2 out]
                n176 = property on="Test Ring" class="Ring (strict)"("Visible"=FALSE) -> ()  [unwired: 2 in, 2 out]
              }
            }
          }
        }
        n177 = property on="Progress" class="Clust (strict)"("Visible"=FALSE) -> ()  [unwired: 2 in, 2 out]
      }
      event "Test Name": Mouse Enter {
        # "Populate the ring with the list of tests"
        n178 = event-data() -> ()  [unwired: 1 in, 1 out]
        n179 = call <vilib>:"NT Read String Array.vi"("Name"="TestMode/TestList") -> ("String Array"=w319:string[])  [unwired: 9 in, 1 out]
        n180 = Build Array (concatenate)("Select the test to run...", w319) -> (w318:string[])
        n181 = property on="Test Name" class="Ring (strict)"("Strings []"=w318) -> ()  [unwired: 2 in, 2 out]
      }
      event "Test Name": Value Change {
        w321 = FALSE ("Visible")
        # "Tell the robot the test name to run"
        n182 = event-data() -> ("NewVal"=w325:u16)  [unwired: 1 in]
        n183 = property on="Test Name" class="Ring (strict)"() -> ("Strings []"=w326:string[])  [unwired: 2 in, 2 out]
        n184 = local write "Progress"(T8 {"Test Progress"=0, "Test Progress Text"=""} ("Progress")) -> ()
        n185 = Index Array(array=w326, index=w325) -> (element=w324:string)
        n186 = call <vilib>:"NT Write String.vi"("String"=w324, "Name"="TestMode/TestName") -> ()  [unwired: 9 in, 1 out]
        n187 = property on="Progress" class="Clust (strict)"("Visible"=TRUE) -> ()  [unwired: 2 in, 2 out]
        n188 = property on="Motor" class="Clust (strict)"("Visible"=w321) -> ()  [unwired: 2 in, 2 out]
        n189 = property on="Test Slider" class="Slide (strict)"("Visible"=w321) -> ()  [unwired: 2 in, 2 out]
        n190 = property on="On/Off" class="Bool (strict)"("Visible"=w321) -> ()  [unwired: 2 in, 2 out]
        n191 = property on="Rev/Fwd" class="Clust (strict)"("Visible"=w321) -> ()  [unwired: 2 in, 2 out]
        n192 = property on="Test Ring" class="Ring (strict)"("Visible"=w321) -> ()  [unwired: 2 in, 2 out]
      }
      event "Listbox": Double Click {
        # "Shift clears all"
        # "Update symbols on the listbox"
        n193 = event-data() -> ("PlatMods.Shift"=w329:bool, "Row"=w331:i32)  [unwired: 1 in]
        n194 = case shown="True" w329 {
          tunnel: w331 -> [w335 _]
          tunnel: 1 -> [w334 _]
          frame False {
            n195 = property on="Listbox" class="LstBox (strict)"() -> ("Item Symbols"=w333:i32[])  [unwired: 2 in, 2 out]
            n196 = Replace Array Subset(array=w333, new element=w334, index=w335) -> (w332:i32[])
            n197 = property on="Listbox" class="LstBox (strict)"("Item Symbols"=w332) -> ()  [unwired: 2 in, 2 out]
          }
          frame True {
            w336 = 0 ("Top Row")
            n198 = property on="Listbox" class="LstBox (strict)"() -> ("Number of Rows"=w338:u32)  [unwired: 2 in, 2 out]
            n199 = Initialize Array(0, w338) -> (w337:i32[])
            n200 = property on="Listbox" class="LstBox (strict)"("Top Row"=w336, "Value"=w336, "Item Symbols"=w337) -> ()  [unwired: 2 in, 2 out]
          }
        }
      }
      event "Listbox": Key Down {
        # "Update symbols on the listbox\nLeft and right keys check and uncheck"
        n201 = event-data() -> ("VKey"=w342:T24)  [unwired: 1 in]
        n202 = case shown="\"Left\", \"Right\"" w342 {
          selector: w342 -> [w347 _]
          tunnel: eventvkey."Left" ("VKey") -> [w345 _]
          frame "Left", "Right" {
            n203 = Equal?(x=w345, y=w347) -> (x = y?=w346:bool)
            n204 = Select(t=0, s=w346, f=1) -> (s? t:f=w348:i32)
            n205 = property on="Listbox" class="LstBox (strict)"() -> ("Item Symbols"=w351:i32[])  [unwired: 2 in, 2 out]
            n206 = Replace Array Subset(array=w351, new element=w348, index="Listbox") -> (w350:i32[])
            n207 = property on="Listbox" class="LstBox (strict)"("Item Symbols"=w350) -> ()  [unwired: 2 in, 2 out]
          }
          frame Default {
          }
        }
      }
      event "DB Camera Config": Value Change {
        # "Show or hide the cluster of controls, store in ini file"
        n208 = event-data() -> ("NewVal"=w355:bool)  [unwired: 1 in]
        n209 = case shown="False" w355 {
          tunnel: w354 -> [w364 _]
          tunnel: [w357 w375] -> w353
          tunnel: w352 -> [w356 w375]
          frame False {
            w371 = "Camera"
            w374 = FALSE ("Visible")
            n210 = local read "Camera Settings"() -> (w363:T3)
            n211 = Index Array(array=w364) -> (element=w367:cluster{string[]})  [unwired: 1 in]
            n212 = Unbundle(w363) -> ("Frame Rate"=w362:i32, "Compression"=w361:i32, "Size"=w365:u16)
            n213 = Unbundle(w367) -> (w366:string[])
            n214 = Index Array(array=w366, index=w365) -> (element=w360:string)
            n215 = call-poly <vilib>:"Write Key.vi"("section"=w371, "value"=w360, "key"="Size", "refnum"=w356) -> ("refnum out"=w373:T22)  [unwired: 2 in, 5 out]
            n216 = call-poly <vilib>:"Write Key.vi"("section"=w371, "value"=w362, "key"="FrameRate", "refnum"=w373) -> ("refnum out"=w372:T22)  [unwired: 1 in, 6 out]
            n217 = property on="Camera Settings" class="Clust (strict)"("Visible"=w374) -> ()  [unwired: 2 in, 2 out]
            n218 = local write "DB Camera Config"(w374) -> ()
            n219 = call-poly <vilib>:"Write Key.vi"("section"=w371, "value"=w361, "key"="Compression", "refnum"=w372) -> ("refnum out"=w358:T22)  [unwired: 1 in, 6 out]
            n220 = call <vilib>:"Close Config Data.vi"("refnum"=w358) -> ("file path"=w359:path)  [unwired: 2 in, 8 out]
            n221 = call <vilib>:"Open Config Data.vi"("configuration file path"=w359) -> ("refnum"=w357:T22)  [unwired: 8 in, 2 out]
          }
          frame True {
            n222 = property on="Camera Settings" class="Clust (strict)"("Visible"=TRUE) -> ()  [unwired: 2 in, 2 out]
          }
        }
      }
      event "Camera Settings": Value Change {
        # "Update summary string when any elements of DB camera change"
        n223 = event-data() -> ("NewVal"=w388:T3)  [unwired: 1 in]
        n224 = Index Array(array=w384) -> (element=w383:cluster{string[]})  [unwired: 1 in]
        n225 = Unbundle(w388) -> ("Frame Rate"=w379:i32, "Compression"=w378:i32, "Size"=w381:u16)
        n226 = Unbundle(w383) -> (w382:string[])
        n227 = Index Array(array=w382, index=w381) -> (element=w380:string)
        n228 = Format Into String(format string="%s   %dfps   %d%%", w380, w379, w378) -> (resulting string=w385:string)  [unwired: 2 in, 1 out]
        n229 = Build Array(w385) -> (w386:string[])
        n230 = property on="DB Camera Config" class="Bool (strict)"("Strings [4]"=w386) -> ()  [unwired: 2 in, 2 out]
      }
      event "Motor.Enable": Value Change {
        # "When the test mode otor enable helper is set, update that\ntree row item's value"
        n231 = event-data() -> ("NewVal"=w394:bool)  [unwired: 1 in]
        n232 = Unbundle("Motor") -> ("Value"=w393:dbl)  [unwired: 1 out]
        n233 = Select(t=w393, s=w394, f=0.0) -> (s? t:f=w391:dbl)
        n234 = call <vilib>:"NT Write Number.vi"("Numeric"=w391, "Name"=w390) -> ()  [unwired: 9 in, 1 out]
      }
      event "Test Slider": Value Change {
        # "When the test mode slider helper is set, update that\ntree row item's value"
        n235 = event-data() -> ("NewVal"=w397:dbl)  [unwired: 1 in]
        n236 = call <vilib>:"NT Write Number.vi"("Numeric"=w397, "Name"=w398) -> ()  [unwired: 9 in, 1 out]
      }
      event "On/Off": Value Change {
        # "When the test mode on/off helper value is set, update that\ntree row item's value"
        n237 = event-data() -> ("NewVal"=w402:bool)  [unwired: 1 in]
        n238 = Boolean To (0,1)(Boolean=w402) -> (0, 1=w401:i16)
        n239 = call <vilib>:"NT Write Number.vi"("Numeric"=w401, "Name"=w400) -> ()  [unwired: 9 in, 1 out]
      }
      event "Rev/Fwd": Value Change {
        # "When the test mode helper value for relays is set, update that\ntree row item's value"
        n240 = event-data() -> ("NewVal.Forward"=w410:bool, "NewVal.Reverse"=w409:bool)  [unwired: 1 in]
        n241 = Boolean To (0,1)(Boolean=w410) -> (0, 1=w406:i16)
        n242 = Boolean To (0,1)(Boolean=w409) -> (0, 1=w408:i16)
        n243 = Negate(x=w408) -> (-x=w407:i16)
        n244 = Add(x=w406, y=w407) -> (x+y=w405:i16)
        n245 = call <vilib>:"NT Write Number.vi"("Numeric"=w405, "Name"=w404) -> ()  [unwired: 9 in, 1 out]
      }
      event "Test Ring": Value Change {
        # "When a test mode helper value is selected from the ring,\nset the tree item's variable to the string value"
        n246 = event-data() -> ("NewVal"=w414:u16)  [unwired: 1 in]
        n247 = property on="Test Ring" class="Ring (strict)"() -> ("Strings []"=w415:string[])  [unwired: 2 in, 2 out]
        n248 = Index Array(array=w415, index=w414) -> (element=w413:string)
        n249 = call <vilib>:"NT Write String.vi"("String"=w413, "Name"=w412) -> ()  [unwired: 9 in, 1 out]
      }
      event "Rec Mode": Value Change {
        # "Update globals for recording mode and path to read log from.\nClear when logging and let NetworkTables set path for vision to\nuse."
        n250 = event-data() -> ("NewVal"=w425:enum32{"Stop", "Record", "Playback"})  [unwired: 1 in]
        n251 = global write "WPI_DashboardLogging Global.vi" "Logging Filename"(path "") -> ()
        n252 = case shown="\"Playback\"" w425 {
          tunnel: w424 -> [_ w427 w435]
          tunnel: [_ _ w434] -> w421
          tunnel: [_ _ w433] -> _
          tunnel: w419 -> [_ _ w431]
          tunnel: cluster{i32, i32} {-250, 170} -> [_ _ w430]
          tunnel: [_ _ T25 {"Image Size"=TRUE, "Image Type"=TRUE, "Pixel Value"=TRUE, "ROI Information"=TRUE, "Zoom Factor"=FALSE} ("Image Information Shown:All Elements")] -> w417
          tunnel: [_ _ TRUE ("Zoom Factor")] -> w416
          frame Default {
          }
          frame "Stop", "Record" {
            # "Place Window too"
            n253 = invoke class="VI" method="FP.Close"(reference=w427) -> (reference out=w426:refnum<vi>)  [unwired: 2 in, 2 out]
            n254 = invoke class="VI" method="Abort VI"(reference=w426) -> ()  [unwired: 2 in, 3 out]
          }
          frame "Playback" {
            n255 = call "Open Playback Panel.vi"("Offset"=w430, "DB VI Ref"=w431, "Playback in"=w435) -> ("Playback out"=w432:refnum<vi>)  [unwired: 8 in]
            n256 = register-events(w432) -> (reference out=w434:refnum<event-registration>, error out=w433:errorcluster)  [unwired: 2 in]
          }
        }
        n257 = global write "WPI_DashboardLogging Global.vi" "Recording"(w425) -> ()
        n258 = property on="Camera Image" class="ImageControl"("Image Information Shown"=w417, "Image Information Visible"=w416) -> ()  [unwired: 2 in, 2 out]
        n259 = call <vilib>:"WPI_DashboardNT Log FieldName Cache.vi"("Operation"=enum16{"Lookup/Add", "Index", "Clear"}."Clear") -> ()  [unwired: 8 in, 3 out]
      }
      event Panel Close {
        w436 = enum32{"Stop", "Record", "Playback"}."Stop" ("Rec Mode")
        # "Playback window has been closed, abort"
        n260 = event-data() -> ()  [unwired: 1 in, 4 out]
        n261 = local write "Rec Mode"(w436) -> ()
        n262 = global write "WPI_DashboardLogging Global.vi" "Recording"(w436) -> ()
      }
      event Panel Close {
        # "Abort playback window and ourself"
        n263 = event-data() -> ()  [unwired: 1 in, 4 out]
        n264 = invoke class="VI" method="FP.Close"(reference=w441) -> (reference out=w440:refnum<vi>)  [unwired: 2 in, 2 out]
        n265 = invoke class="VI" method="Abort VI"(reference=w440) -> (error out=w439:errorcluster)  [unwired: 2 in, 2 out]
        n266 = invoke class="VI" method="Abort VI"(error in=w439) -> ()  [unwired: 2 in, 3 out]
      }
      event "Vision": Value Change {
        # "Enable/Disable Compression slider.\nHW USB is hard-coded into the camera"
        n267 = event-data() -> ("NewVal"=w447:u16)  [unwired: 1 in]
        n268 = Equal?(x=w447, y=u32 2 ("milliseconds to wait")) -> (x = y?=w445:bool)
        n269 = Select(t=T26."Disabled and Grayed Out" ("Disabled"), s=w445, f=T26."Enabled" ("Disabled")) -> (s? t:f=w442:T26)
        n270 = property on="Compression" class="Slide (strict)"("DisabledEnum"=w442) -> ()  [unwired: 2 in, 2 out]
      }
    }
  }
  n271 = call "readMotorPodConfig.vi"("Input Pod Clustor"=w31, "Pod Number"=1, "Refnum in"=w22) -> ("Pod Output"=w27:T10)  [unwired: 6 in]
  n272 = call "readMotorPodConfig.vi"("Input Pod Clustor"=w30, "Pod Number"=2, "Refnum in"=w22) -> ("Pod Output"=w26:T10)  [unwired: 6 in]
  n273 = call "readMotorPodConfig.vi"("Input Pod Clustor"=w29, "Pod Number"=3, "Refnum in"=w22) -> ("Pod Output"=w24:T10)  [unwired: 6 in]
  n274 = call "readMotorPodConfig.vi"("Input Pod Clustor"=w28, "Pod Number"=4, "Refnum in"=w22) -> ("Pod Output"=w25:T10)  [unwired: 6 in]
  n275 = while {
    tunnel: w84 -> [w450]
    i -> [w453]
    stop <- FALSE stop-if-true
    n276 = Wait (ms)(milliseconds to wait=u32 100) -> ()  [unwired: 1 out]
    n277 = case shown="\"Playback\"" "Rec Mode" {
      tunnel: w453 -> [_ _ w468]
      tunnel: [u32 2829099 ("Base Color") u32 11141120 ("Target Color") w457] -> w449
      frame "Stop", Default {
        # "Reset the color, extra updates don't cost much"
      }
      frame "Record" {
      }
      frame "Playback" {
        # "Playback"
        n278 = Quotient & Remainder(x=w468, y=u32 50 ("milliseconds to wait")) -> (x-y*floor(x/y)=w464:u32)  [unwired: 1 out]
        n279 = Divide(x=w464, y=u32 50 ("milliseconds to wait")) -> (x/y=w461:dbl)
        n280 = Multiply(x=6.283185307179586, y=w461) -> (x*y=w466:dbl)
        n281 = Sine(x=w466) -> (sin(x)=w465:dbl)
        n282 = Absolute Value(x=w465) -> (abs(x)=w458:dbl)
        n283 = call "Interpolate RGB Color.vi"("Proportion"=w458, "Target Color"=u32 30976, "Base Color"=u32 2829099) -> ("Result Color"=w457:u32)  [unwired: 8 in]
      }
    }
    n284 = property class="Pane"(reference=w450, "PaneColor"=w449) -> ()  [unwired: 1 in, 2 out]
  }
  n285 = global write "Config_Global.vi" "Pod 0"(w27) -> ()
  n286 = global write "Config_Global.vi" "Pod 1"(w26) -> ()
  n287 = global write "Config_Global.vi" "Pod 2"(w24) -> ()
  n288 = global write "Config_Global.vi" "Pod 3"(w25) -> ()
  n289 = global read "Config_Global.vi" "Pod 0"() -> (w21:T10)
  n290 = global read "Config_Global.vi" "Pod 1"() -> (w20:T10)
  n291 = global read "Config_Global.vi" "Pod 2"() -> (w19:T10)
  n292 = global read "Config_Global.vi" "Pod 3"() -> (w18:T10)
  n293 = call "readMotorPodTurret.vi"("Input Pod Clustor"=w21, "Pod Number"=1, "Refnum in"=w22) -> ("output cluster"=w17:T10)  [unwired: 6 in]
  n294 = call "readMotorPodTurret.vi"("Input Pod Clustor"=w20, "Pod Number"=2, "Refnum in"=w22) -> ("output cluster"=w16:T10)  [unwired: 6 in]
  n295 = call "readMotorPodTurret.vi"("Input Pod Clustor"=w19, "Pod Number"=3, "Refnum in"=w22) -> ("output cluster"=w15:T10)  [unwired: 6 in]
  n296 = call "readMotorPodTurret.vi"("Input Pod Clustor"=w18, "Pod Number"=4, "Refnum in"=w22) -> ("output cluster"=w14:T10)  [unwired: 6 in]
  n297 = TCP Create Listener(10:u16 1741 ("timeout ms (25000)")) -> (3:w47:refnum<k5>)  [unwired: 4 in, 2 out]
  n298 = global write "Config_Global.vi" "Pod 0"(w17) -> ()
  n299 = global write "Config_Global.vi" "Pod 1"(w16) -> ()
  n300 = global write "Config_Global.vi" "Pod 2"(w15) -> ()
  n301 = global write "Config_Global.vi" "Pod 3"(w14) -> ()
  n302 = while {
    tunnel: w47 -> [w470]
    stop <- FALSE stop-if-true
    n303 = TCP Wait On Listener(11:w470) -> (4:w469:refnum<k5>)  [unwired: 3 in, 4 out]
    n304 = local write "TCP"(w469) -> ()
  }
  n305 = global read "Config_Global.vi" "Pod 0"() -> (w13:T10)
  n306 = global read "Config_Global.vi" "Pod 1"() -> (w12:T10)
  n307 = global read "Config_Global.vi" "Pod 2"() -> (w11:T10)
  n308 = global read "Config_Global.vi" "Pod 3"() -> (w10:T10)
  n309 = property on="On/Off" class="Bool (strict)"("Visible"=w52) -> ()  [unwired: 2 in, 2 out]
  n310 = property on="Motor" class="Clust (strict)"("Visible"=w52) -> ()  [unwired: 2 in, 2 out]
  n311 = property on="Progress" class="Clust (strict)"("Visible"=w52) -> ()  [unwired: 2 in, 2 out]
  n312 = property on="Test Ring" class="Ring (strict)"("Visible"=w52) -> ()  [unwired: 2 in, 2 out]
  n313 = property on="Rev/Fwd" class="Clust (strict)"("Visible"=w52) -> ()  [unwired: 2 in, 2 out]
  n314 = call "readMotorPodMisc.vi"("Input Pod Clustor"=w13, "Pod Number"=1, "Refnum in"=w22) -> ("output cluster"=w9:T10)  [unwired: 8 in]
  n315 = call "readMotorPodMisc.vi"("Input Pod Clustor"=w12, "Pod Number"=2, "Refnum in"=w22) -> ("output cluster"=w8:T10)  [unwired: 8 in]
  n316 = call "readMotorPodMisc.vi"("Input Pod Clustor"=w11, "Pod Number"=3, "Refnum in"=w22) -> ("output cluster"=w7:T10)  [unwired: 8 in]
  n317 = call "readMotorPodMisc.vi"("Input Pod Clustor"=w10, "Pod Number"=4, "Refnum in"=w22) -> ("output cluster"=w6:T10)  [unwired: 8 in]
  n318 = property on="Camera Settings" class="Clust (strict)"("Visible"=w52) -> ()  [unwired: 2 in, 2 out]
  n319 = local write "DB Camera Config"(w52) -> ()
  n320 = global write "Config_Global.vi" "Pod 0"(w9) -> ()
  n321 = global write "Config_Global.vi" "Pod 1"(w8) -> ()
  n322 = global write "Config_Global.vi" "Pod 2"(w7) -> ()
  n323 = global write "Config_Global.vi" "Pod 3"(w6) -> ()
  n324 = global write "WPI_DashboardLogging Global.vi" "Recording"(w78) -> ()
  n325 = local write "Rec Mode"(w78) -> ()
  n326 = call <vilib>:"Close Config Data.vi"("error in (no error)"=w23, "refnum"=w22) -> ("error out"=→"error out":errorcluster)  [unwired: 8 in, 1 out]
  n327 = global read "Config_Global.vi" "Pod 0"() -> (w5:T10)
  n328 = global read "Config_Global.vi" "Pod 1"() -> (w2:T10)
  n329 = global read "Config_Global.vi" "Pod 2"() -> (w4:T10)
  n330 = global read "Config_Global.vi" "Pod 3"() -> (w3:T10)
  n331 = global read "Config_Global.vi" "General"() -> (w1:T11)
  n332 = local write "General"(w1) -> ()
  n333 = local write "Pod 0"(w5) -> ()
  n334 = local write "Pod 1"(w2) -> ()
  n335 = local write "Pod 2"(w4) -> ()
  n336 = local write "Pod 3"(w3) -> ()
  n337 = event shown="[2] \"Pod 1\": Value Change" {
    selector: _ -> [_ _ _ _ _]
    dyn-events: _ -> [_ _ _ _ _]
    timeout: _ -> [_ _ _ _ _]
    event Timeout {
      # "Listens for user input on front panel"
      n338 = event-data() -> ()  [unwired: 1 in, 3 out]
    }
    event "Pod 0": Value Change {
      w478 = 0  # Pod Number
      # "Listens for user input on front panel"
      n339 = event-data() -> ("NewVal"=w486:T10)  [unwired: 1 in]
      n340 = Unbundle By Name(w486) -> ("Drive"=w485:T28, "Turret"=w481:T29, "Misc"=w479:T30)
      n341 = call <vilib>:"Open Config Data.vi"("configuration file path"=path "C:/Users/Developer/Documents/LabVIEW Data/2016 Dashboard (adam)/ConfigData/configData.ini" ("local path")) -> ("refnum"=w483:T22)  [unwired: 8 in, 2 out]
      n342 = call "writeDrive.vi"("Pod Number"=w478, "Drive"=w485, "Refnum in"=w483) -> ("error out"=w475:errorcluster, "Refnum in 2"=w482:T22)  [unwired: 7 in]
      n343 = call "writeTurret.vi"("error in (no error)"=w475, "Turret"=w481, "Pod Number"=w478, "Refnum in"=w482) -> ("error out"=w474:errorcluster, "Refnum out"=w480:T22)  [unwired: 6 in]
      n344 = call "writeMisc.vi"("error in (no error)"=w474, "Misc"=w479, "Pod Number"=w478, "Refnum in"=w480) -> ("error out"=w477:errorcluster, "Refnum out"=w476:T22)  [unwired: 6 in]
      n345 = call <vilib>:"Close Config Data.vi"("error in (no error)"=w477, "write file if changed (T)"=TRUE, "refnum"=w476) -> ("error out"=→"error out":errorcluster)  [unwired: 7 in, 1 out]
    }
    event "Pod 1": Value Change {
      w495 = 1  # Pod Number
      # "Listens for user input on front panel"
      n346 = event-data() -> ("NewVal"=w487:T10)  [unwired: 1 in]
      n347 = Unbundle By Name(w487) -> ("Drive"=w489:T28, "Turret"=w492:T29, "Misc"=w494:T30)
      n348 = call <vilib>:"Open Config Data.vi"("configuration file path"=path "C:/Users/Developer/Documents/LabVIEW Data/2016 Dashboard (adam)/ConfigData/configData.ini" ("local path")) -> ("refnum"=w490:T22)  [unwired: 8 in, 2 out]
      n349 = call "writeDrive.vi"("Pod Number"=w495, "Drive"=w489, "Refnum in"=w490) -> ("error out"=w498:errorcluster, "Refnum in 2"=w491:T22)  [unwired: 7 in]
      n350 = call "writeTurret.vi"("error in (no error)"=w498, "Turret"=w492, "Pod Number"=w495, "Refnum in"=w491) -> ("error out"=w499:errorcluster, "Refnum out"=w493:T22)  [unwired: 6 in]
      n351 = call "writeMisc.vi"("error in (no error)"=w499, "Misc"=w494, "Pod Number"=w495, "Refnum in"=w493) -> ("error out"=w496:errorcluster, "Refnum out"=w497:T22)  [unwired: 6 in]
      n352 = call <vilib>:"Close Config Data.vi"("error in (no error)"=w496, "write file if changed (T)"=TRUE, "refnum"=w497) -> ("error out"=→"error out 2":errorcluster)  [unwired: 7 in, 1 out]
    }
    event "Pod 2": Value Change {
      w510 = 2  # Pod Number
      # "Listens for user input on front panel"
      n353 = event-data() -> ("NewVal"=w503:T10)  [unwired: 1 in]
      n354 = Unbundle By Name(w503) -> ("Drive"=w516:T28, "Turret"=w513:T29, "Misc"=w511:T30)
      n355 = call <vilib>:"Open Config Data.vi"("configuration file path"=path "C:/Users/Developer/Documents/LabVIEW Data/2016 Dashboard (adam)/ConfigData/configData.ini" ("local path")) -> ("refnum"=w515:T22)  [unwired: 8 in, 2 out]
      n356 = call "writeDrive.vi"("Pod Number"=w510, "Drive"=w516, "Refnum in"=w515) -> ("error out"=w507:errorcluster, "Refnum in 2"=w514:T22)  [unwired: 7 in]
      n357 = call "writeTurret.vi"("error in (no error)"=w507, "Turret"=w513, "Pod Number"=w510, "Refnum in"=w514) -> ("error out"=w506:errorcluster, "Refnum out"=w512:T22)  [unwired: 6 in]
      n358 = call "writeMisc.vi"("error in (no error)"=w506, "Misc"=w511, "Pod Number"=w510, "Refnum in"=w512) -> ("error out"=w509:errorcluster, "Refnum out"=w508:T22)  [unwired: 6 in]
      n359 = call <vilib>:"Close Config Data.vi"("error in (no error)"=w509, "write file if changed (T)"=TRUE, "refnum"=w508) -> ("error out"=→"error out 3":errorcluster)  [unwired: 7 in, 1 out]
    }
    event "Pod 3": Value Change {
      w525 = 3  # Pod Number
      # "Listens for user input on front panel"
      n360 = event-data() -> ("NewVal"=w517:T10)  [unwired: 1 in]
      n361 = Unbundle By Name(w517) -> ("Drive"=w531:T28, "Turret"=w528:T29, "Misc"=w526:T30)
      n362 = call <vilib>:"Open Config Data.vi"("configuration file path"=path "C:/Users/Developer/Documents/LabVIEW Data/2016 Dashboard (adam)/ConfigData/configData.ini" ("local path")) -> ("refnum"=w530:T22)  [unwired: 8 in, 2 out]
      n363 = call "writeDrive.vi"("Pod Number"=w525, "Drive"=w531, "Refnum in"=w530) -> ("error out"=w522:errorcluster, "Refnum in 2"=w529:T22)  [unwired: 7 in]
      n364 = call "writeTurret.vi"("error in (no error)"=w522, "Turret"=w528, "Pod Number"=w525, "Refnum in"=w529) -> ("error out"=w521:errorcluster, "Refnum out"=w527:T22)  [unwired: 6 in]
      n365 = call "writeMisc.vi"("error in (no error)"=w521, "Misc"=w526, "Pod Number"=w525, "Refnum in"=w527) -> ("error out"=w524:errorcluster, "Refnum out"=w523:T22)  [unwired: 6 in]
      n366 = call <vilib>:"Close Config Data.vi"("error in (no error)"=w524, "write file if changed (T)"=TRUE, "refnum"=w523) -> ("error out"=→"error out 4":errorcluster)  [unwired: 7 in, 1 out]
    }
  }
